vi "TEST - Reverse 2D Array.vi"(8 "error in (no error)":errorcluster) -> (0 "error out":errorcluster, 2 "Pass?":bool=TRUE)   [LabVIEW 2020]
doc: "This VI template can be used for the functional testing of VIs; this implementation includes handling for the testing of polymorphic VIs, and the polymorphic elements should be removed if not needed.\n\nCoded by Douglas A. Femec, January 24, 2006.\n\nCopyright (c) 2005-2006 MKS Instruments, Inc.\nAll rights reserved."
uses:
  TEST - Reverse 2D Array - Inputs.ctl
  Polymorphizer+ Data Type.ctl
  TEST - Reverse 2D Array - Outputs.ctl
  source/library/Reverse 2D Array/Reverse 2D Array (EXT).vi
  source/library/Reverse 2D Array/Reverse 2D Array (I64).vi
  source/library/Reverse 2D Array/Reverse 2D Array (U64).vi
  source/library/Reverse 2D Array/Reverse 2D Array (LVObject).vi
  source/library/Reverse 2D Array/Reverse 2D Array (DBL).vi
  source/library/Reverse 2D Array/Reverse 2D Array (SGL).vi
  source/library/Reverse 2D Array/Reverse 2D Array (I32).vi
  source/library/Reverse 2D Array/Reverse 2D Array (I16).vi
  source/library/Reverse 2D Array/Reverse 2D Array (I8).vi
  source/library/Reverse 2D Array/Reverse 2D Array (U32).vi
  source/library/Reverse 2D Array/Reverse 2D Array (U16).vi
  source/library/Reverse 2D Array/Reverse 2D Array (U8).vi
  source/library/Reverse 2D Array/Reverse 2D Array (CXT).vi
  source/library/Reverse 2D Array/Reverse 2D Array (CDB).vi
  source/library/Reverse 2D Array/Reverse 2D Array (CSG).vi
  source/library/Reverse 2D Array/Reverse 2D Array (Boolean).vi
  source/library/Reverse 2D Array/Reverse 2D Array (String).vi
  source/library/Reverse 2D Array/Reverse 2D Array (Path).vi
  source/library/Reverse 2D Array/Reverse 2D Array (Variant).vi
  TestClass/TestClass.lvclass
panel:
  out "Generated Outputs":T1[][](array[typedef]) {"2D Array" format="%.2f"}
  in  "Expected Outputs":T1[](array[typedef])=[{"Description"="Expect empty array", "2D Array"=[]}, {"Description"="Expect empty array", "2D Array"=[]}, {"Description"="Expect 1D row", "2D Array"=[[1.0], [1.0], [0.0], [1.0], [0.0]]}, {"Description"="Expect 1D row", "2D Array"=[[0.0], [1.0], [0.0], [1.0], [1.0]]}, {"Description"="Expect 1D column", "2D Array"=[[1.0, 0.0]]}, {"Description"="Expect 1D column", "2D Array"=[[0.0, 1.0]]}, {"Description"="Expect 2D array", "2D Array"=[[1.0, 0.0], [1.0, 0.0], [0.0, 1.0], [1.0, 0.0], [0.0, 1.0]]}, {"Description"="Expect 2D array", "2D Array"=[[1.0, 0.0], [0.0, 1.0], [1.0, 0.0], [0.0, 1.0], [0.0, 1.0]]}] {"2D Array" format="%.2f"}
  in  "Inputs":T2[](array[typedef])=[{"Description"="Empty array, by rows", "Data Types to Test"=[enum."EXT", enum."DBL", enum."SGL", enum."I32", enum."I16", enum."I8", enum."U32", enum."U16", enum."U8", enum."CXT", enum."CDB", enum."CSG", enum."Boolean", enum."String", enum."Path", enum."Variant", enum."LabVIEW Object", enum."I64", enum."U64"], "2D Array"=[], "by rows or columns (rows)"=enum."rows"}, {"Description"="Empty array, by columns", "Data Types to Test"=[enum."EXT", enum."DBL", enum."SGL", enum."I32", enum."I16", enum."I8", enum."U32", enum."U16", enum."U8", enum."CXT", enum."CDB", enum."CSG", enum."Boolean", enum."String", enum."Path", enum."Variant", enum."LabVIEW Object", enum."I64", enum."U64"], "2D Array"=[], "by rows or columns (rows)"=enum."columns"}, {"Description"="1D row, by rows", "Data Types to Test"=[enum."EXT", enum."DBL", enum."SGL", enum."I32", enum."I16", enum."I8", enum."U32", enum."U16", enum."U8", enum."CXT", enum."CDB", enum."CSG", enum."Boolean", enum."String", enum."Path", enum."Variant", enum."LabVIEW Object", enum."I64", enum."U64"], "2D Array"=[[0.0], [1.0], [0.0], [1.0], [1.0]], "by rows or columns (rows)"=enum."rows"}, {"Description"="1D row, by columns", "Data Types to Test"=[enum."EXT", enum."DBL", enum."SGL", enum."I32", enum."I16", enum."I8", enum."U32", enum."U16", enum."U8", enum."CXT", enum."CDB", enum."CSG", enum."Boolean", enum."String", enum."Path", enum."Variant", enum."LabVIEW Object", enum."I64", enum."U64"], "2D Array"=[[0.0], [1.0], [0.0], [1.0], [1.0]], "by rows or columns (rows)"=enum."columns"}, {"Description"="1D column, by rows", "Data Types to Test"=[enum."EXT", enum."DBL", enum."SGL", enum."I32", enum."I16", enum."I8", enum."U32", enum."U16", enum."U8", enum."CXT", enum."CDB", enum."CSG", enum."Boolean", enum."String", enum."Path", enum."Variant", enum."LabVIEW Object", enum."I64", enum."U64"], "2D Array"=[[1.0, 0.0]], "by rows or columns (rows)"=enum."rows"}, {"Description"="1D column, by columns", "Data Types to Test"=[enum."EXT", enum."DBL", enum."SGL", enum."I32", enum."I16", enum."I8", enum."U32", enum."U16", enum."U8", enum."CXT", enum."CDB", enum."CSG", enum."Boolean", enum."String", enum."Path", enum."Variant", enum."LabVIEW Object", enum."I64", enum."U64"], "2D Array"=[[1.0, 0.0]], "by rows or columns (rows)"=enum."columns"}, {"Description"="2D array, by rows", "Data Types to Test"=[enum."EXT", enum."DBL", enum."SGL", enum."I32", enum."I16", enum."I8", enum."U32", enum."U16", enum."U8", enum."CXT", enum."CDB", enum."CSG", enum."Boolean", enum."String", enum."Path", enum."Variant", enum."LabVIEW Object", enum."I64", enum."U64"], "2D Array"=[[0.0, 1.0], [1.0, 0.0], [0.0, 1.0], [1.0, 0.0], [1.0, 0.0]], "by rows or columns (rows)"=enum."rows"}, {"Description"="2D array, by columns", "Data Types to Test"=[enum."EXT", enum."DBL", enum."SGL", enum."I32", enum."I16", enum."I8", enum."U32", enum."U16", enum."U8", enum."CXT", enum."CDB", enum."CSG", enum."String", enum."Path", enum."LabVIEW Object", enum."I64", enum."U64"], "2D Array"=[[0.0, 1.0], [1.0, 0.0], [0.0, 1.0], [1.0, 0.0], [1.0, 0.0]], "by rows or columns (rows)"=enum."columns"}] {"2D Array" format="%.2f"}
  # "Copyright (c) 2005-2006 MKS Instruments, Inc.\nAll rights reserved."
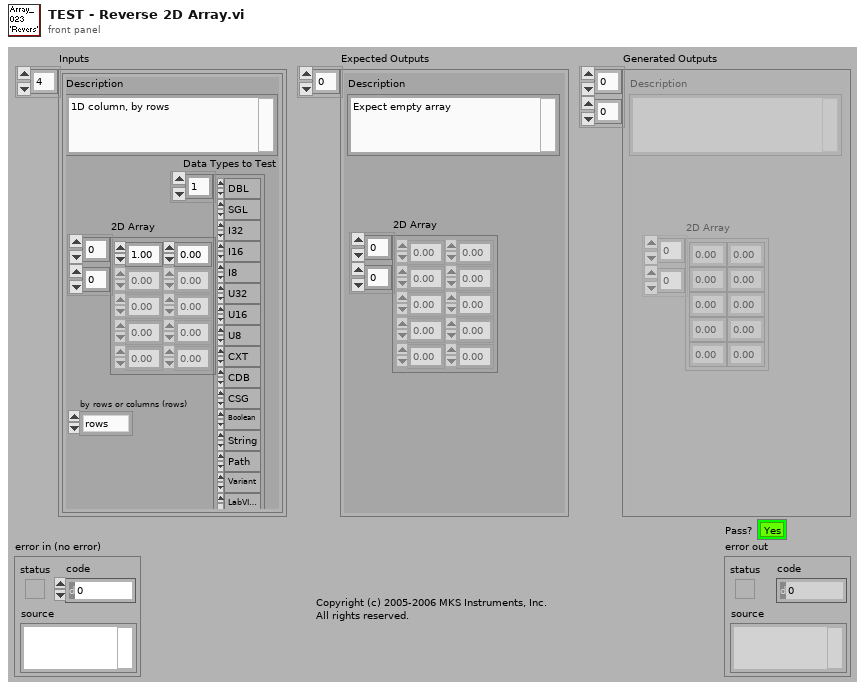
[diagram p1: front panel]
types:
  T1 = typedef "TEST - Reverse 2D Array - Outputs.ctl" = cluster{"Description":string, "2D Array":sgl[][]}
  T2 = typedef "TEST - Reverse 2D Array - Inputs.ctl" = cluster{"Description":string, "Data Types to Test":T3[], "2D Array":sgl[][], "by rows or columns (rows)":enum16{"rows", "columns"}}
  T3 = typedef "Polymorphizer+ Data Type.ctl" = enum16{"EXT", "DBL", "SGL", "I32", "I16", "I8", "U32", "U16", "U8", "CXT", "CDB", "CSG", "Boolean", "String", "Path", "Variant", "CTL-REF", "GEN-REF", "GObj-REF", "VI-REF", "ENUM", "ERR", "FILE-REF", "MENU-REF", "MENU-RING", "PICT-RING", "TXT&PICT-RING", "TXT-RING", "I64", "U64", "LabVIEW Object"}
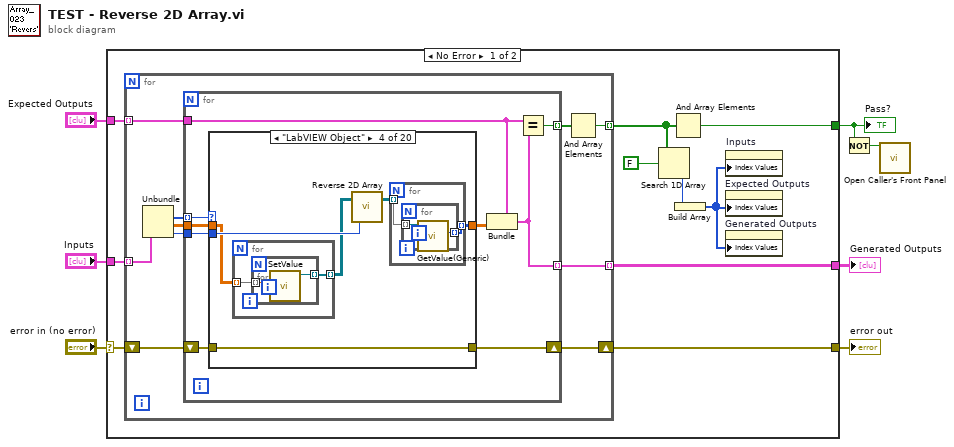
[diagram p0: block diagram]
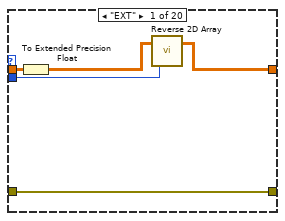
[diagram p2: hidden frame]
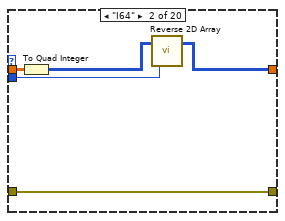
[diagram p3: hidden frame]
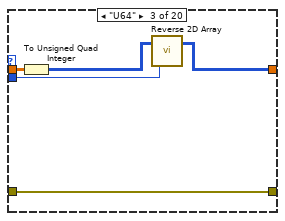
[diagram p4: hidden frame]
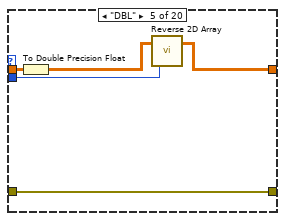
[diagram p5: hidden frame]
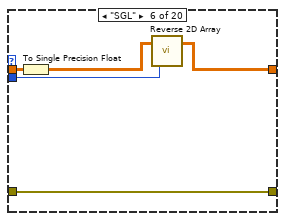
[diagram p6: hidden frame]
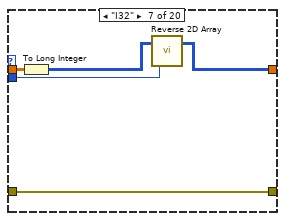
[diagram p7: hidden frame]
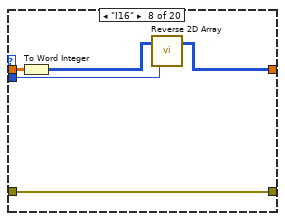
[diagram p8: hidden frame]
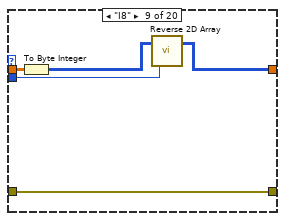
[diagram p9: hidden frame]
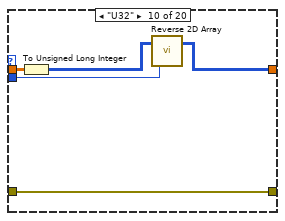
[diagram p10: hidden frame]
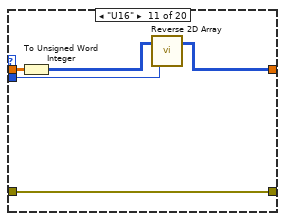
[diagram p11: hidden frame]
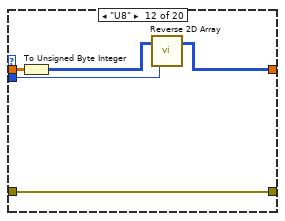
[diagram p12: hidden frame]
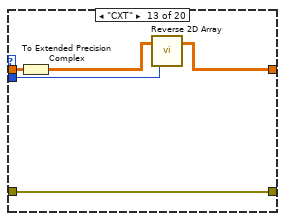
[diagram p13: hidden frame]
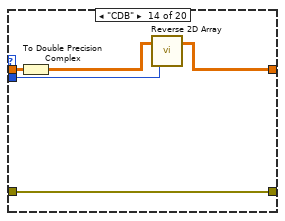
[diagram p14: hidden frame]
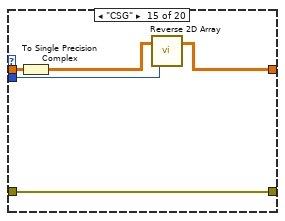
[diagram p15: hidden frame]
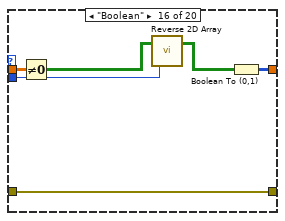
[diagram p16: hidden frame]
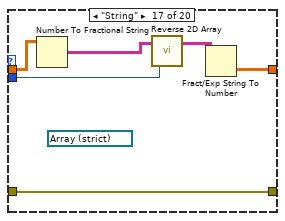
[diagram p17: hidden frame]
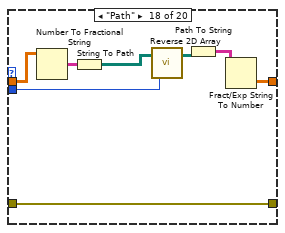
[diagram p18: hidden frame]
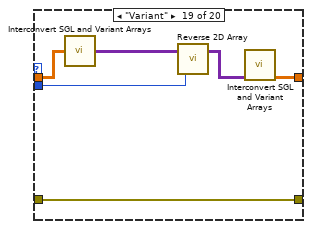
[diagram p19: hidden frame]
diagram:
  n1 = case shown="No Error" "error in (no error)" {
    selector: "error in (no error)" -> [w16 w149]
    tunnel: [w17 w149] -> w6
    tunnel: "Expected Outputs" -> [w14 _]
    tunnel: "Inputs" -> [w15 _]
    tunnel: [w13 _] -> w3
    tunnel: [w12 _] -> w1
    frame No Error {
      n2 = for {
        shift-right: [w22] -> w17
        shift-left: w16 -> [w23]
        tunnel: w15 -> [w24] mode=indexing
        tunnel: w14 -> [w27] mode=indexing
        tunnel: [w26] -> w13 mode=indexing
        tunnel: [w21] -> w11 mode=indexing
        n3 = Unbundle(w24) -> ("Data Types to Test"=w20:T3[], "2D Array"=w19:sgl[][], "by rows or columns (rows)"=w18:enum16{"rows", "columns"})  [unwired: 1 out]
        n4 = for {
          tunnel: w27 -> [w36]
          tunnel: [w34] -> w26 mode=indexing
          tunnel: [w35] -> w25 mode=indexing
          shift-right: [w30] -> w22
          shift-left: w23 -> [w31]
          tunnel: w20 -> [w32] mode=indexing
          tunnel: w19 -> [w33]
          tunnel: w18 -> [w28]
          n5 = case shown="\"LabVIEW Object\"" w32 {
            tunnel: w33 -> [w41 w46 w51 w55 w70 w75 w80 w85 w90 w95 w100 w105 w110 w115 w120 w126 w132 w139 w144 w147]
            tunnel: [w38 w43 w48 w52 w67 w71 w76 w81 w86 w91 w96 w101 w106 w111 w116 w123 w129 w137 w142 w147] -> w29
            tunnel: w31 -> [w40 w45 w50 w57 w69 w74 w79 w84 w89 w94 w99 w104 w109 w114 w119 w125 w131 w138 w146 w148]
            tunnel: [w40 w45 w50 w57 w69 w74 w79 w84 w89 w94 w99 w104 w109 w114 w119 w125 w131 w138 w146 w148] -> w30
            tunnel: w28 -> [w37 w42 w47 w56 w66 w72 w77 w82 w87 w92 w97 w102 w107 w112 w117 w124 w128 w135 w145 _]
            frame "EXT" {
              n6 = To Extended Precision Float(1:w41) -> (0:w39:ext[][])
              n7 = call-poly "Reverse 2D Array.vi"("by rows or columns (rows)"=w37, "Array"=w39) -> ("Reversed Array"=w38:ext[][])  [unwired: 1 in]
            }
            frame "I64" {
              n8 = To Quad Integer(1:w46) -> (0:w44:i64[][])
              n9 = call-poly "Reverse 2D Array.vi"("by rows or columns (rows)"=w42, "Array"=w44) -> ("Reversed Array"=w43:i64[][])  [unwired: 1 in]
            }
            frame "U64" {
              n10 = To Unsigned Quad Integer(1:w51) -> (0:w49:u64[][])
              n11 = call-poly "Reverse 2D Array.vi"("by rows or columns (rows)"=w47, "Array"=w49) -> ("Reversed Array"=w48:u64[][])  [unwired: 1 in]
            }
            frame "LabVIEW Object" {
              n12 = for {
                tunnel: w55 -> [w63] mode=indexing
                tunnel: [w62] -> w54 mode=indexing
                n13 = for {
                  tunnel: w63 -> [w65] mode=indexing
                  tunnel: [w64] -> w62 mode=indexing
                  n14 = call "SetValue.vi"("Value"=w65) -> ("TestClass out"=w64:refnum<class "TestClass.lvclass">)  [unwired: 9 in, 1 out]
                }
              }
              n15 = call-poly "Reverse 2D Array.vi"("by rows or columns (rows)"=w56, "Array"=w54) -> ("Reversed Array"=w53:refnum<class>[][])  [unwired: 1 in]
              n16 = for {
                tunnel: w53 -> [w59] mode=indexing
                tunnel: [w58] -> w52 mode=indexing
                n17 = for {
                  tunnel: w59 -> [w60] mode=indexing
                  tunnel: [w61] -> w58 mode=indexing
                  n18 = call "GetValue(Generic).vi"("TestClass in"=w60) -> ("Value"=w61:i32)  [unwired: 8 in, 2 out]
                }
              }
            }
            frame "DBL" {
              n19 = To Double Precision Float(number=w70) -> (double precision float=w68:dbl[][])
              n20 = call-poly "Reverse 2D Array.vi"("by rows or columns (rows)"=w66, "Array"=w68) -> ("Reversed Array"=w67:dbl[][])  [unwired: 1 in]
            }
            frame "SGL" {
              n21 = To Single Precision Float(number=w75) -> (single precision float=w73:sgl[][])
              n22 = call-poly "Reverse 2D Array.vi"("by rows or columns (rows)"=w72, "Array"=w73) -> ("Reversed Array"=w71:sgl[][])  [unwired: 1 in]
            }
            frame "I32" {
              n23 = To Long Integer(number=w80) -> (32bit integer=w78:i32[][])
              n24 = call-poly "Reverse 2D Array.vi"("by rows or columns (rows)"=w77, "Array"=w78) -> ("Reversed Array"=w76:i32[][])  [unwired: 1 in]
            }
            frame "I16" {
              n25 = To Word Integer(number=w85) -> (16bit integer=w83:i16[][])
              n26 = call-poly "Reverse 2D Array.vi"("by rows or columns (rows)"=w82, "Array"=w83) -> ("Reversed Array"=w81:i16[][])  [unwired: 1 in]
            }
            frame "I8" {
              n27 = To Byte Integer(number=w90) -> (8bit integer=w88:i8[][])
              n28 = call-poly "Reverse 2D Array.vi"("by rows or columns (rows)"=w87, "Array"=w88) -> ("Reversed Array"=w86:i8[][])  [unwired: 1 in]
            }
            frame "U32" {
              n29 = To Unsigned Long Integer(number=w95) -> (unsigned 32bit integer=w93:u32[][])
              n30 = call-poly "Reverse 2D Array.vi"("by rows or columns (rows)"=w92, "Array"=w93) -> ("Reversed Array"=w91:u32[][])  [unwired: 1 in]
            }
            frame "U16" {
              n31 = To Unsigned Word Integer(number=w100) -> (unsigned 16bit integer=w98:u16[][])
              n32 = call-poly "Reverse 2D Array.vi"("by rows or columns (rows)"=w97, "Array"=w98) -> ("Reversed Array"=w96:u16[][])  [unwired: 1 in]
            }
            frame "U8" {
              n33 = To Unsigned Byte Integer(number=w105) -> (unsigned 8bit integer=w103:u8[][])
              n34 = call-poly "Reverse 2D Array.vi"("by rows or columns (rows)"=w102, "Array"=w103) -> ("Reversed Array"=w101:u8[][])  [unwired: 1 in]
            }
            frame "CXT" {
              n35 = To Extended Precision Complex(1:w110) -> (0:w108:cxt[][])
              n36 = call-poly "Reverse 2D Array.vi"("by rows or columns (rows)"=w107, "Array"=w108) -> ("Reversed Array"=w106:cxt[][])  [unwired: 1 in]
            }
            frame "CDB" {
              n37 = To Double Precision Complex(1:w115) -> (0:w113:cdb[][])
              n38 = call-poly "Reverse 2D Array.vi"("by rows or columns (rows)"=w112, "Array"=w113) -> ("Reversed Array"=w111:cdb[][])  [unwired: 1 in]
            }
            frame "CSG" {
              n39 = To Single Precision Complex(1:w120) -> (0:w118:csg[][])
              n40 = call-poly "Reverse 2D Array.vi"("by rows or columns (rows)"=w117, "Array"=w118) -> ("Reversed Array"=w116:csg[][])  [unwired: 1 in]
            }
            frame "Boolean" {
              n41 = Not Equal To 0?(x=w126) -> (x != 0?=w122:bool[][])
              n42 = call-poly "Reverse 2D Array.vi"("by rows or columns (rows)"=w124, "Array"=w122) -> ("Reversed Array"=w121:bool[][])  [unwired: 1 in]
              n43 = Boolean To (0,1)(Boolean=w121) -> (0, 1=w123:i16[][])
            }
            frame "String" {
              (unwired) refnum<vi> refnum ("Inputs")
              n44 = Number To Fractional String(number=w132) -> (F-format string=w130:string[][])  [unwired: 3 in]
              n45 = call-poly "Reverse 2D Array.vi"("by rows or columns (rows)"=w128, "Array"=w130) -> ("Reversed Array"=w127:string[][])  [unwired: 1 in]
              n46 = Fract/Exp String To Number(string=w127) -> (number=w129:dbl[][])  [unwired: 3 in, 1 out]
            }
            frame "Path" {
              n47 = Number To Fractional String(number=w139) -> (F-format string=w140:string[][])  [unwired: 3 in]
              n48 = String To Path(string=w140) -> (path=w134:path[][])
              n49 = call-poly "Reverse 2D Array.vi"("by rows or columns (rows)"=w135, "Array"=w134) -> ("Reversed Array"=w133:path[][])  [unwired: 1 in]
              n50 = Path To String(path=w133) -> (string=w136:string[][])
              n51 = Fract/Exp String To Number(string=w136) -> (number=w137:dbl[][])  [unwired: 3 in, 1 out]
            }
            frame "Variant" {
              n52 = call "Interconvert SGL and Variant Arrays.vi"("SGL 2D Array In"=w144) -> ("Variant 2D Array Out"=w143:variant[][])  [unwired: 10 in, 4 out]
              n53 = call-poly "Reverse 2D Array.vi"("by rows or columns (rows)"=w145, "Array"=w143) -> ("Reversed Array"=w141:variant[][])  [unwired: 1 in]
              n54 = call "Interconvert SGL and Variant Arrays.vi"("Variant 2D Array In"=w141) -> ("SGL 2D Array Out"=w142:sgl[][])  [unwired: 10 in, 4 out]
            }
            frame Default {
            }
          }
          n55 = Bundle(cluster=w36, "2D Array"=w29) -> (w34:T1)  [unwired: 1 in]
          n56 = Equal?(x=w36, y=w34) -> (x = y?=w35:bool)
        }
        n57 = And Array Elements(Boolean array=w25) -> (logical AND=w21:bool)
      }
      n58 = Search 1D Array(1D array=w11, element=FALSE) -> (index of element=w9:i32)  [unwired: 1 in]
      n59 = And Array Elements(Boolean array=w11) -> (logical AND=w12:bool)
      n60 = Build Array(w9) -> (w8:i32[])
      n61 = property on="Inputs" class="Arr (strict)"("Index Values"=w8) -> ()  [unwired: 2 in, 2 out]
      n62 = property on="Expected Outputs" class="Arr (strict)"("Index Values"=w8) -> ()  [unwired: 2 in, 2 out]
      n63 = property on="Generated Outputs" class="Arr (strict)"("Index Values"=w8) -> ()  [unwired: 2 in, 2 out]
    }
    frame Error {
    }
  }
  "error out" <- w6
  "Pass?" <- w1
  "Generated Outputs" <- w3
  n64 = Not(x=w1) -> (.not. x?=w2:bool)
  n65 = call "Open Caller's Front Panel.vi"("Open?"=w2) -> ()  [unwired: 14 in, 1 out]
